vi "ExperimentType.vi"(8 "error in (no error)":errorcluster, 11 "TrialBasedExperiment in":refnum<class "TrialBasedExperiment.lvclass">) -> (0 "error out":errorcluster, 2 "Params":T1={"PassiveTask"=FALSE, "AcquireFixation"=TRUE, "CanStop"=TRUE, "MustStop"=FALSE}, 3 "TrialBasedExperiment out":refnum<class "TrialBasedExperiment.lvclass">)   [LabVIEW 2010]
uses:
  TrialBasedExperiment.lvclass
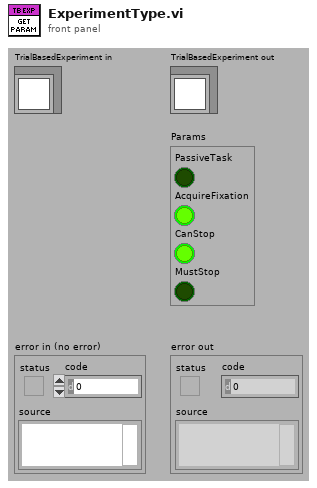
[diagram p1: front panel]
types:
  T1 = cluster{"PassiveTask":bool, "AcquireFixation":bool, "CanStop":bool, "MustStop":bool}
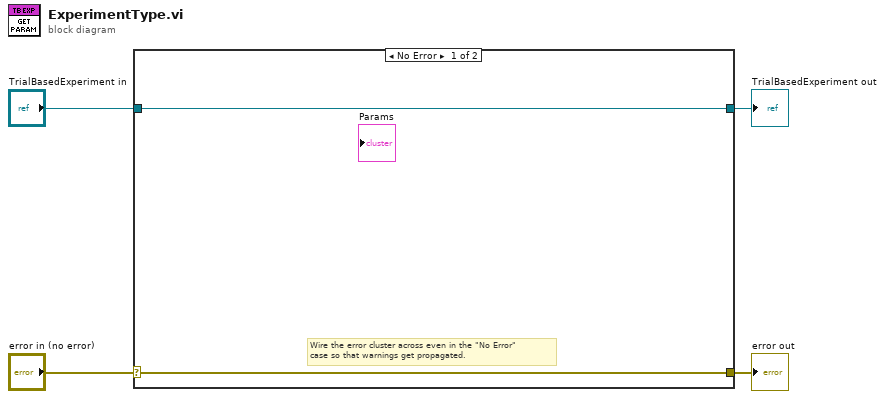
[diagram p0: block diagram]
diagram:
  n1 = case shown="No Error" "error in (no error)" {
    selector: "error in (no error)" -> [w5 w8]
    tunnel: [w5 w8] -> w3
    tunnel: [w6 w7] -> w1
    tunnel: "TrialBasedExperiment in" -> [w6 w7]
    frame No Error {
      # "Wire the error cluster across even in the \"No Error\"\ncase so that warnings get propagated."
    }
    frame Error {
    }
  }
  "error out" <- w3
  "TrialBasedExperiment out" <- w1
